vi "UI.vi"(8 "error in (no error)":errorcluster) -> (0 "error out":errorcluster)   [LabVIEW 2018]
doc: "SubVI criada para gerenciamento da interface de usuário"
uses:
  Support VIs/Globals.vi
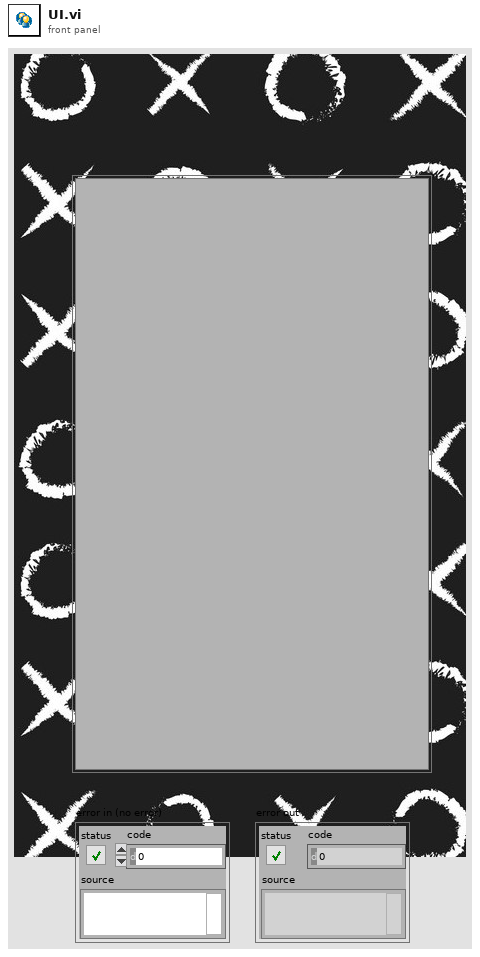
[diagram p1: front panel]
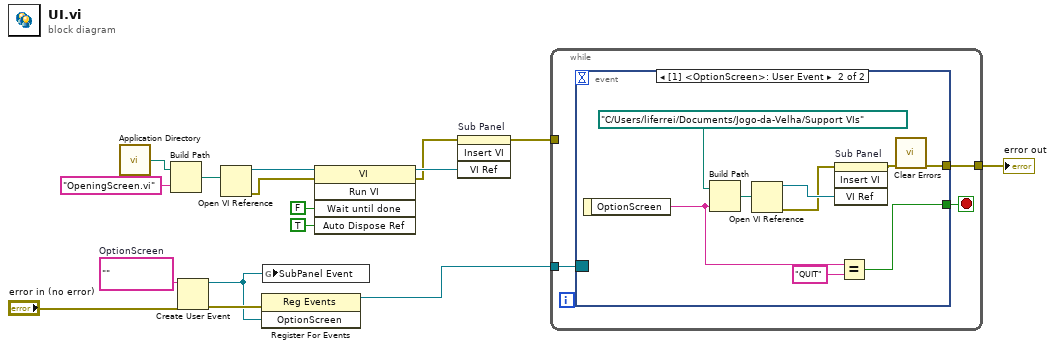
[diagram p0: block diagram]
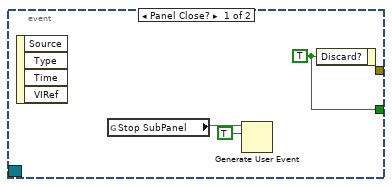
[diagram p2: hidden frame]
diagram:
  w4 = ""  # OptionScreen
  n1 = call <vilib>:"Application Directory.vi"() -> ("Application Directory"=w16:path)
  n2 = Build Path(base path=w16, name or relative path="OpeningScreen.vi") -> (appended path=w14:path)
  n3 = Create User Event(user event datatype=w4, error in="error in (no error)") -> (user event=w2:refnum<user-event>, error out=w3:errorcluster)
  n4 = Open VI Reference(vi path=w14) -> (vi reference=w13:refnum<vi>, error out=w9:errorcluster)  [unwired: 5 in]
  n5 = register-events(error in=w3, w2) -> (reference out=w7:refnum<event-registration>)  [unwired: 1 in, 1 out]
  n6 = global write "Globals.vi" "SubPanel Event"(w2) -> ()
  n7 = invoke class="VI" method="Run VI"(reference=w13, error in=w9, "Wait until done"=FALSE ("Wait Until Done"), "Auto Dispose Ref"=TRUE ("Auto Dispose Reference")) -> (reference out=w12:refnum<vi>, error out=w8:errorcluster)  [unwired: 1 in, 3 out]
  n8 = invoke on="Sub Panel" class="SubPnl" method="Insert VI"(error in=w8, "VI Ref"=w12) -> (error out=w1:errorcluster)  [unwired: 2 in, 3 out]
  n9 = while {
    tunnel: w1 -> [_]
    tunnel: w7 -> [w18]
    tunnel: [w17] -> w5
    stop <- w19 stop-if-true
    n10 = event shown="[1] <OptionScreen>: User Event" {
      selector: w18 -> [_ _]
      dyn-events: _ -> [_ _]
      timeout: _ -> [_ _]
      tunnel: [w22 w27] -> w19
      tunnel: [_ w24] -> w17
      event Panel Close? {
        w22 = TRUE ("Discard?")
        n11 = event-data() -> ()  [unwired: 1 in, 4 out]
        n12 = global read "Globals.vi" "Stop SubPanel"() -> (w21:refnum<user-event>)
        n13 = Generate User Event(user event=w21, event data cluster=TRUE ("event data")) -> ()  [unwired: 2 in, 2 out]
        n14 = event-data("Discard?"=w22) -> ()  [unwired: 1 in, 1 out]
      }
      event User Event {
        n15 = event-data() -> ("OptionScreen"=w29:string)  [unwired: 1 in]
        n16 = Build Path(base path=path "C:/Users/liferrei/Documents/Jogo-da-Velha/Support VIs", name or relative path=w29) -> (appended path=w31:path)
        n17 = Open VI Reference(vi path=w31) -> (vi reference=w30:refnum<vi>, error out=w25:errorcluster)  [unwired: 5 in]
        n18 = invoke on="Sub Panel" class="SubPnl" method="Insert VI"(error in=w25, "VI Ref"=w30) -> (error out=w26:errorcluster)  [unwired: 2 in, 3 out]
        n19 = Equal?(x=w29, y="QUIT") -> (x = y?=w27:bool)
        n20 = call <vilib>:"Clear Errors.vi"("error in (no error)"=w26) -> ("error out"=w24:errorcluster)  [unwired: 5 in, 1 out]
      }
    }
  }
  "error out" <- w5
